vi "DIO - Enable Digital Output.vi"(8 "error in":errorcluster, 10 "Channel Number":i32, 11 "TCP Network Connection in":refnum<k5>) -> (0 "error out":errorcluster, 3 "TCP Network Connection out":refnum<k5>)   [LabVIEW 2020]
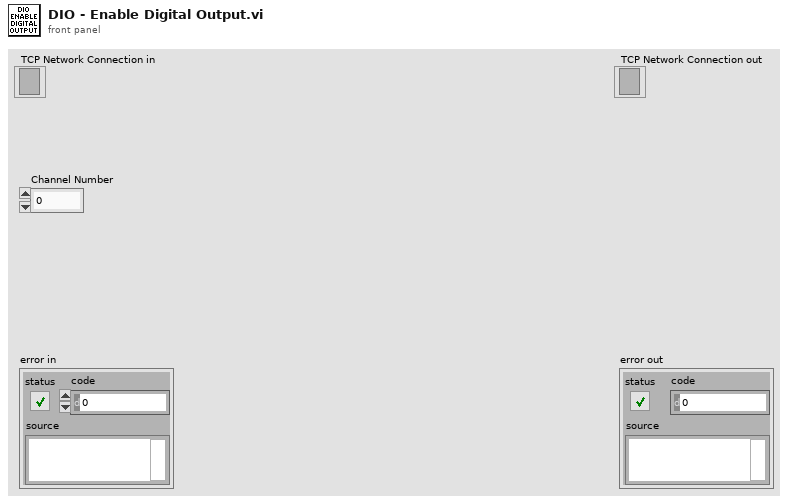
[diagram p1: front panel]
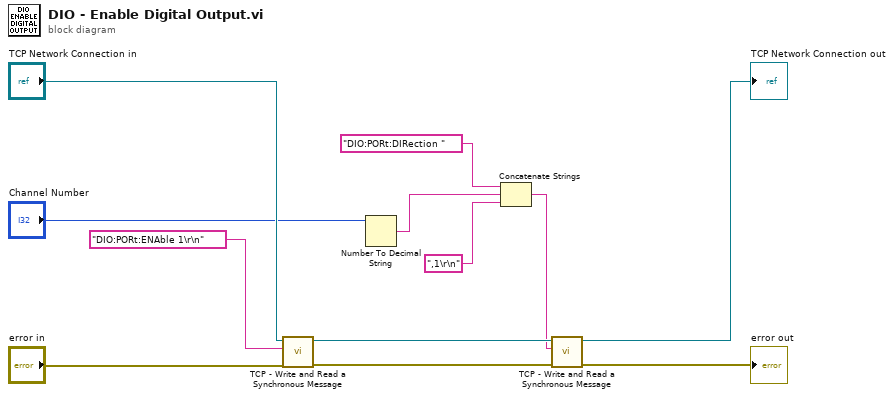
[diagram p0: block diagram]
diagram:
  n1 = call "TCP - Write and Read a Synchronous Message.vi"("error in"="error in", "Message to Send"="DIO:PORt:ENAble 1\r\n", "TCP Network Connection in"="TCP Network Connection in") -> ("error out"=w8:errorcluster, "TCP Network Connection out"=w9:refnum<k5>)  [unwired: 6 in, 1 out]
  n2 = Number To Decimal String(number="Channel Number") -> (decimal integer string=w3:string)  [unwired: 1 in]
  n3 = Concatenate Strings("DIO:PORt:DIRection " ("Message to Send"), w3, ",1\r\n" ("string")) -> (w5:string)
  n4 = call "TCP - Write and Read a Synchronous Message.vi"("error in"=w8, "Message to Send"=w5, "TCP Network Connection in"=w9) -> ("error out"=→"error out":errorcluster, "TCP Network Connection out"=→"TCP Network Connection out":refnum<k5>)  [unwired: 6 in, 1 out]
